vi "Automatic-parking-main.vi"() -> ()   [LabVIEW 2023]
uses:
  subVI/GlobalValues.vi
panel:
  in  "Error In":errorcluster
  out "wrzucona kwota":string
  in  "OK":bool caption="ZATWIERDZ"
  in  "Wprowadz rejestracje":string
  out "output array":string[](array[string])
  in  "input array":string[](array[string])
  in  "zaparkuj":bool
  in  "odbierz":bool
  in  "start":bool
  in  "stop":bool
  # "Wpłacono:"
  # "Cennik:\n12,50 zł - pierwsza godzina\n17 gr - każda kolejna minuta (10,20/h)"
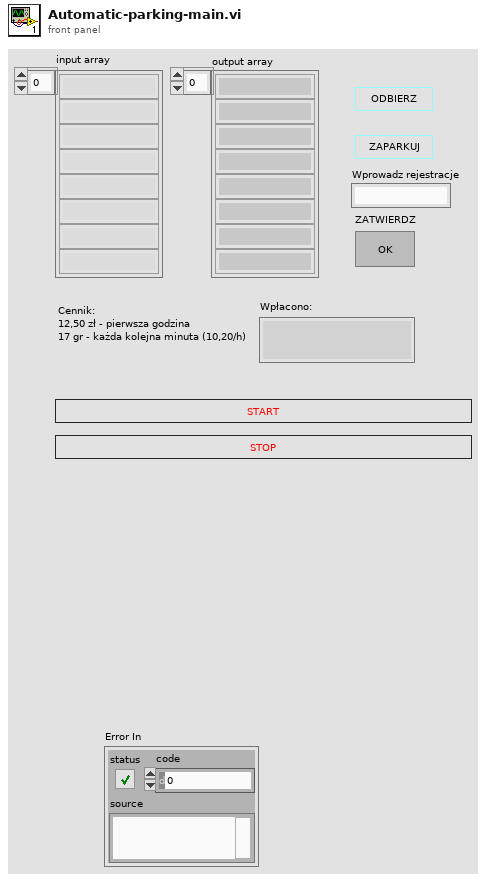
[diagram p1: front panel]
types:
  T1 = enum16{"oczekiwanie", "start", "wpisywanie rejestracji1", "wpisywanie rejestracji2", "zaplata za 1h", "wyjazd z parkingu", "wjazd auta", "doplata"}
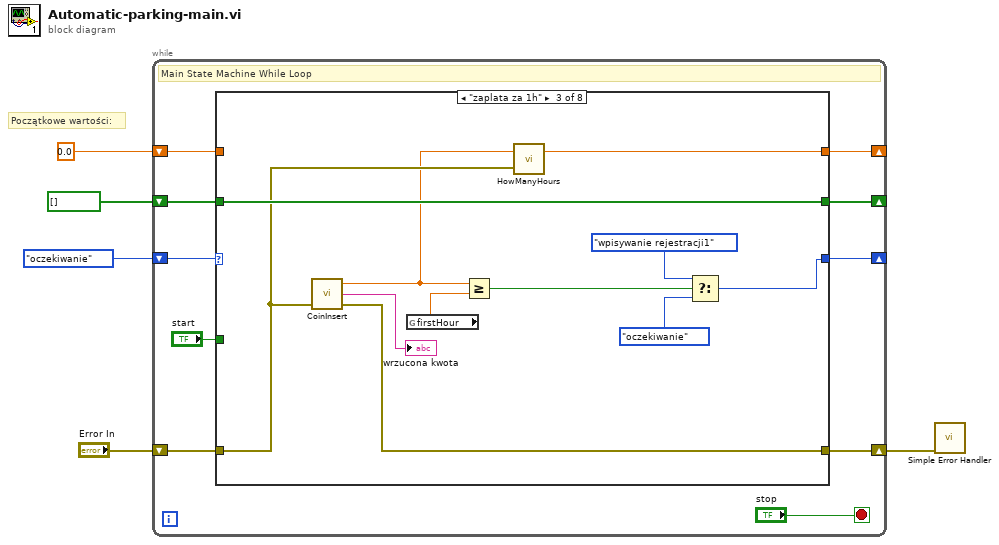
[diagram p0: block diagram]
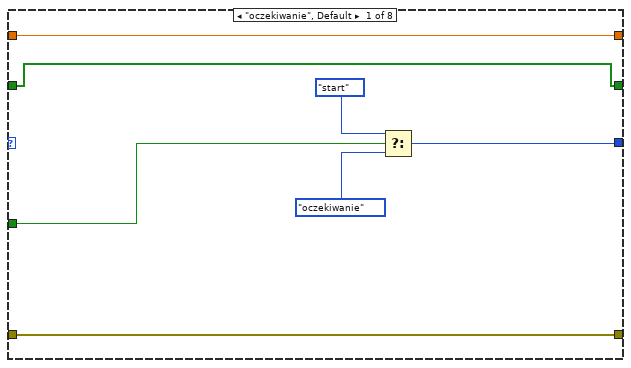
[diagram p2: hidden frame]
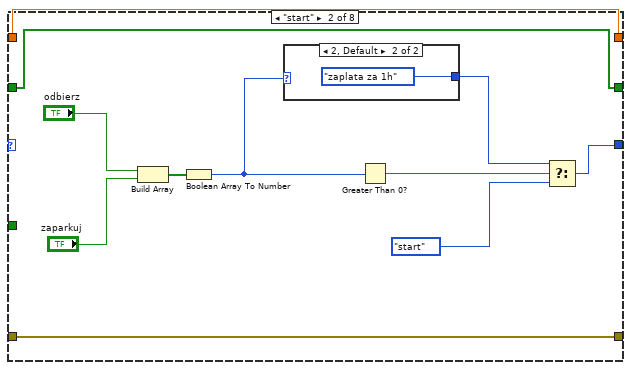
[diagram p3: hidden frame]
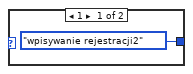
[diagram p4: hidden frame]
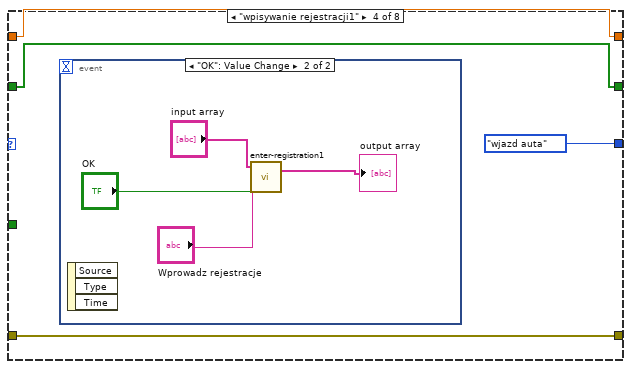
[diagram p5: hidden frame]
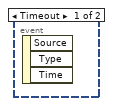
[diagram p6: hidden frame]
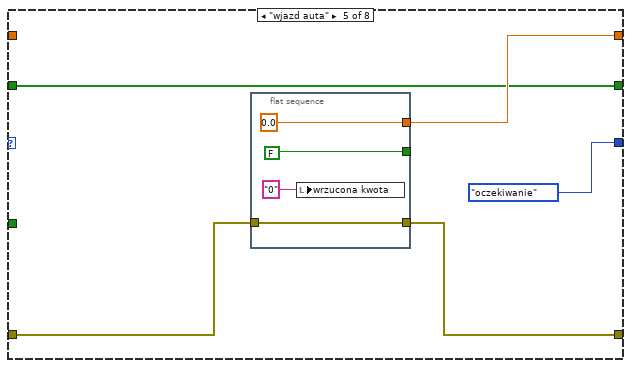
[diagram p7: hidden frame]
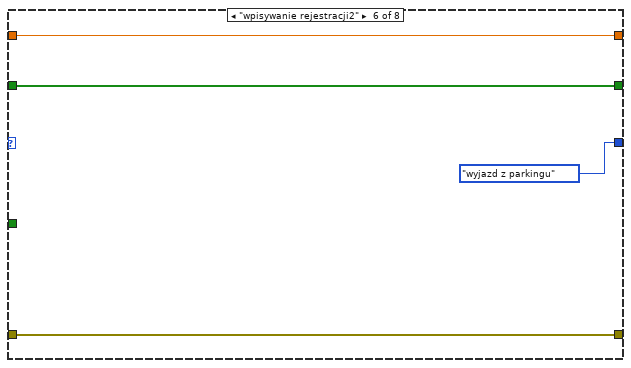
[diagram p8: hidden frame]
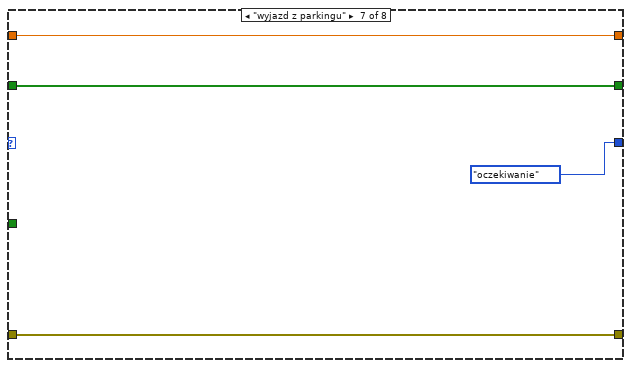
[diagram p9: hidden frame]
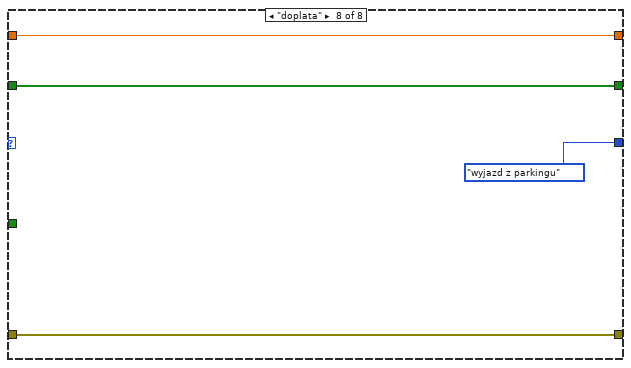
[diagram p10: hidden frame]
diagram:
  # "Początkowe wartości:"
  n1 = while {
    shift-right: [w13] -> _
    shift-left: T1."oczekiwanie" -> [w14]
    shift-right: [w11] -> w4
    shift-left: "Error In" -> [w10]
    shift-right: [w8] -> _
    shift-left: 0.0 -> [w9]
    shift-right: [w6] -> _
    shift-left: bool[] [] -> [w7]
    stop <- "stop" stop-if-true
    # "Main State Machine While Loop"
    n2 = case shown="\"zaplata za 1h\"" w14 {
      tunnel: [w22 w31 w39 T1."wjazd auta" T1."oczekiwanie" T1."wyjazd z parkingu" T1."oczekiwanie" T1."wyjazd z parkingu"] -> w13
      tunnel: "start" -> [w21 _ _ _ _ _ _ _]
      tunnel: [w18 w25 w43 w49 w57 w66 w70 w74] -> w11
      tunnel: w10 -> [w18 w25 w37 w49 w58 w66 w70 w74]
      tunnel: [w16 w23 w41 w47 w55 w64 w68 w72] -> w6
      tunnel: w9 -> [w17 w24 _ w48 _ w65 w69 w73]
      tunnel: [w17 w24 w38 w48 w56 w65 w69 w73] -> w8
      tunnel: w7 -> [w16 w23 w41 w47 w55 w64 w68 w72]
      frame "oczekiwanie", Default {
        n3 = Select(t=T1."start", s=w21, f=T1."oczekiwanie") -> (s? t:f=w22:T1)
      }
      frame "start" {
        n4 = Build Array("odbierz", "zaparkuj") -> (w30:bool[])
        n5 = Boolean Array To Number(Boolean array=w30) -> (number=w27:u32)
        n6 = case shown="2, Default" w27 {
          tunnel: [T1."wpisywanie rejestracji2" T1."zaplata za 1h"] -> w28
          frame 1 {
          }
          frame 2, Default {
          }
        }
        n7 = Greater Than 0?(x=w27) -> (x > 0?=w29:bool)
        n8 = Select(t=w28, s=w29, f=T1."start") -> (s? t:f=w31:T1)
      }
      frame "zaplata za 1h" {
        n9 = call "CoinInsert.vi"("Error In"=w37) -> ("Error Out"=w43:errorcluster, "wrzucona kwota"=→"wrzucona kwota":string, "Numeric"=w36:dbl)  [unwired: 2 in]
        n10 = global read "GlobalValues.vi" "firstHour"() -> (w40:dbl)
        n11 = Greater Or Equal?(x=w36, y=w40) -> (x >= y?=w42:bool)
        n12 = call "HowManyHours.vi"("Error In"=w37, "Money"=w36) -> ("MoneyToGo"=w38:dbl)  [unwired: 1 out]
        n13 = Select(t=T1."wpisywanie rejestracji1", s=w42, f=T1."oczekiwanie") -> (s? t:f=w39:T1)
      }
      frame "wpisywanie rejestracji1" {
        n14 = event shown="[1] \"OK\": Value Change" {
          selector: _ -> [_ _]
          dyn-events: _ -> [_ _]
          timeout: _ -> [_ _]
          event Timeout {
            n15 = event-data() -> ()  [unwired: 1 in, 3 out]
          }
          event "OK": Value Change {
            n16 = event-data() -> ()  [unwired: 1 in, 3 out]
            n17 = call "enter-registration1.vi"("OK"="OK", "registration"="Wprowadz rejestracje", "input array"="input array") -> ("output array"=→"output array":string[])
          }
        }
      }
      frame "wjazd auta" {
        n18 = flat-sequence {
          tunnel: w58 -> [w63]
          tunnel: [w63] -> w57
          tunnel: [FALSE] -> _
          tunnel: [0.0] -> w56
          frame #0 {
            n19 = local write "wrzucona kwota"("0" ("Cash")) -> ()
          }
        }
      }
      frame "wpisywanie rejestracji2" {
      }
      frame "wyjazd z parkingu" {
      }
      frame "doplata" {
      }
    }
  }
  n20 = call <vilib>:"Simple Error Handler.vi"("error in (no error)"=w4) -> ()  [unwired: 4 in, 5 out]
